vi "Write My Data to Binary.vi"(4 "Data":T1(array[cluster]), 5 "Comment":string, 7 "Time Stamp":timestamp, 8 "error in":errorcluster, 11 "file path":path) -> (0 "error out":errorcluster)   [LabVIEW 2011]
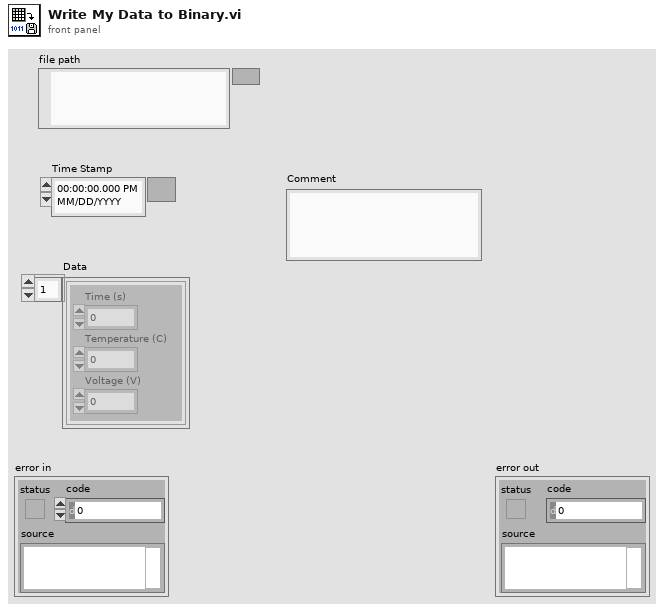
[diagram p1: front panel]
types:
  T1 = cluster{"Time (s)":dbl, "Temperature (C)":dbl, "Voltage (V)":dbl}[]
  T2 = enum16{"open", "replace", "create", "open or create", "replace or create", "replace or create with confirmation"}
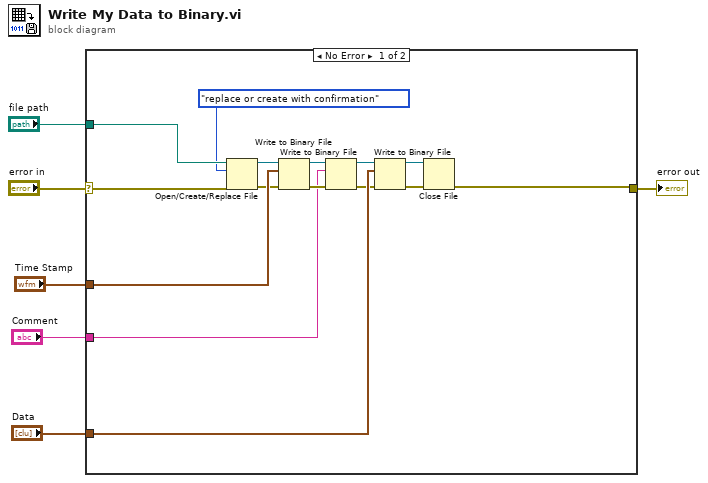
[diagram p0: block diagram]
diagram:
  n1 = case shown="No Error" "error in" {
    selector: "error in" -> [w20 w22]
    tunnel: "Data" -> [w12 _]
    tunnel: [w7 w22] -> w6
    tunnel: "file path" -> [w21 _]
    tunnel: "Time Stamp" -> [w17 _]
    tunnel: "Comment" -> [w13 _]
    frame No Error {
      n2 = Open/Create/Replace File(file path (use dialog)=w21, error in=w20, operation (0:open)=T2."replace or create with confirmation") -> (refnum out=w18:refnum<file>, error out=w16:errorcluster)  [unwired: 3 in, 1 out]
      n3 = Write to Binary File(file (use dialog)=w18, data=w17, error in=w16) -> (refnum out=w14:refnum<file>, error out=w15:errorcluster)  [unwired: 3 in, 1 out]
      n4 = Write to Binary File(file (use dialog)=w14, data=w13, error in=w15) -> (refnum out=w10:refnum<file>, error out=w11:errorcluster)  [unwired: 3 in, 1 out]
      n5 = Write to Binary File(file (use dialog)=w10, data=w12, error in=w11) -> (refnum out=w8:refnum<file>, error out=w9:errorcluster)  [unwired: 3 in, 1 out]
      n6 = Close File(refnum=w8, error in=w9) -> (error out=w7:errorcluster)  [unwired: 1 out]
    }
    frame Error {
      # "Wire previous error through"
    }
  }
  "error out" <- w6
